vi "NanotecSMCPD.convert status.vi"(1 "status":T1 items=["motorEnabled"=1, "negativeLimitSwitchActive"=2, "positiveLimitSwitchActive"=4, "limitSwitchesEnabled"=8, "limitSwitchesAreNormallyClosed"=16, "moving"=32, "referenced"=64, "inPosition"=128, "reserved2"=256, "reserved3"=512, "reserved4"=1024, "reserved5"=2048, "error"=4096, "reserved6"=8192, "reserved7"=16384, "reserved8"=32768, "user defined1"=65536, "user defined2"=131072, "user defined3"=262144, "user defined4"=524288, "user defined5"=1048576, "user defined6"=2097152, "user defined7"=4194304, "user defined8"=8388608, "user defined9"=16777216, "user defined10"=33554432, "user defined11"=67108864, "user defined12"=134217728, "user defined13"=268435456, "user defined14"=536870912, "user defined15"=1073741824, "user defined16"=2147483648], 2 "actStatus type":T2) -> (15 "status out":T1 items=["motorEnabled"=1, "negativeLimitSwitchActive"=2, "positiveLimitSwitchActive"=4, "limitSwitchesEnabled"=8, "limitSwitchesAreNormallyClosed"=16, "moving"=32, "referenced"=64, "inPosition"=128, "reserved2"=256, "reserved3"=512, "reserved4"=1024, "reserved5"=2048, "error"=4096, "reserved6"=8192, "reserved7"=16384, "reserved8"=32768, "user defined1"=65536, "user defined2"=131072, "user defined3"=262144, "user defined4"=524288, "user defined5"=1048576, "user defined6"=2097152, "user defined7"=4194304, "user defined8"=8388608, "user defined9"=16777216, "user defined10"=33554432, "user defined11"=67108864, "user defined12"=134217728, "user defined13"=268435456, "user defined14"=536870912, "user defined15"=1073741824, "user defined16"=2147483648], 16 "motorOn":bool)   [LabVIEW 2014, in "NanotecSMCPD.lvlib"]
doc: "converts the status bytes received from the instrument driver to 32bit status word used by the MotorBase class."
uses:
  NanotecSMCPD.lvlib
  CSinstr.lib/NanotecSMCPD/Public/Action-Status/NanotecSMCPDDriver.status type.ctl
  CSCore/CSApplicationBaseClasses/MotorBase/MotorBase.statusType.ctl
  CSCore/CSApplicationBaseClasses/MotorBase/MotorBase.lvlib
  CSinstr.lib/NanotecSMCPD/NanotecSMCPDDriver.lvlib
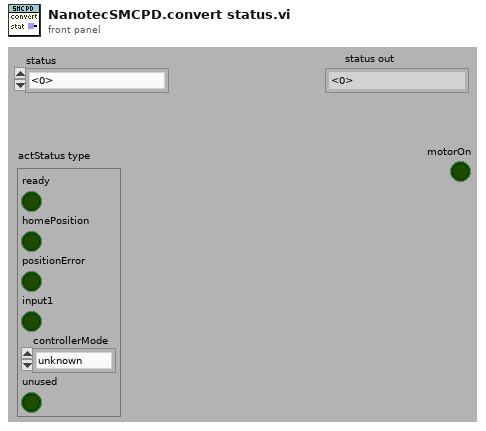
[diagram p1: front panel]
types:
  T1 = typedef "MotorBase.lvlib/MotorBase.statusType.ctl" = u32
  T2 = typedef "NanotecSMCPDDriver.lvlib/NanotecSMCPDDriver.status type.ctl" = cluster{"ready":bool, "homePosition":bool, "positionError":bool, "input1":bool, "controllerMode":enum16{"unknown", "position", "speed", "flagPosition", "clockDirection", "analog", "joystick", "unused"}, "unused":bool}
  T3 = enum16{"unknown", "position", "speed", "flagPosition", "clockDirection", "analog", "joystick", "unused"}
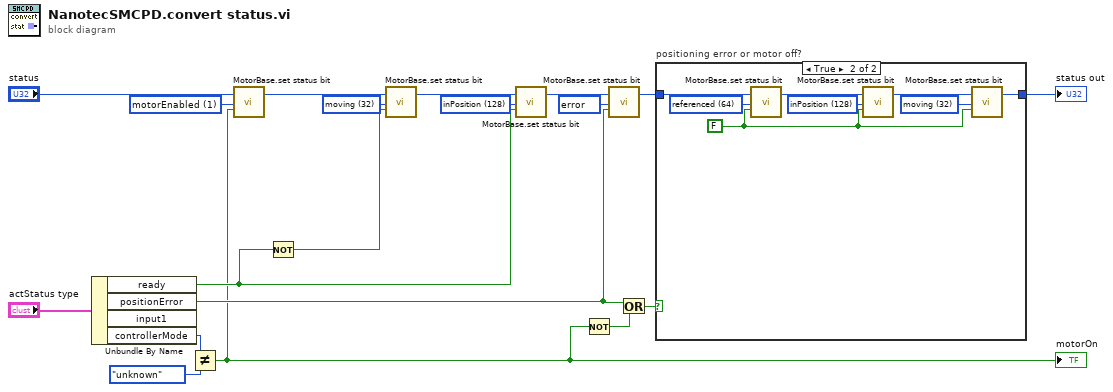
[diagram p0: block diagram]
diagram:
  w8 = T1 32 items=["motorEnabled"=1, "negativeLimitSwitchActive"=2, "positiveLimitSwitchActive"=4, "limitSwitchesEnabled"=8, "limitSwitchesAreNormallyClosed"=16, "moving"=32, "referenced"=64, "inPosition"=128, "reserved2"=256, "reserved3"=512, "reserved4"=1024, "reserved5"=2048, "error"=4096, "reserved6"=8192, "reserved7"=16384, "reserved8"=32768, "user defined1"=65536, "user defined2"=131072, "user defined3"=262144, "user defined4"=524288, "user defined5"=1048576, "user defined6"=2097152, "user defined7"=4194304, "user defined8"=8388608, "user defined9"=16777216, "user defined10"=33554432, "user defined11"=67108864, "user defined12"=134217728, "user defined13"=268435456, "user defined14"=536870912, "user defined15"=1073741824, "user defined16"=2147483648] ("statusBit")
  w15 = T1 4096 items=["motorEnabled"=1, "negativeLimitSwitchActive"=2, "positiveLimitSwitchActive"=4, "limitSwitchesEnabled"=8, "limitSwitchesAreNormallyClosed"=16, "reseved1"=32, "referenced"=64, "inPosition"=128, "reserved2"=256, "reserved3"=512, "reserved4"=1024, "reserved5"=2048, "error"=4096, "reserved6"=8192, "reserved7"=16384, "reserved8"=32768, "user defined1"=65536, "user defined2"=131072, "user defined3"=262144, "user defined4"=524288, "user defined5"=1048576, "user defined6"=2097152, "user defined7"=4194304, "user defined8"=8388608, "user defined9"=16777216, "user defined10"=33554432, "user defined11"=67108864, "user defined12"=134217728, "user defined13"=268435456, "user defined14"=536870912, "user defined15"=1073741824, "user defined16"=2147483648] ("statusBit")
  w16 = T1 128 items=["motorEnabled"=1, "negativeLimitSwitchActive"=2, "positiveLimitSwitchActive"=4, "limitSwitchesEnabled"=8, "limitSwitchesAreNormallyClosed"=16, "reseved1"=32, "referenced"=64, "inPosition"=128, "reserved2"=256, "reserved3"=512, "reserved4"=1024, "reserved5"=2048, "error"=4096, "reserved6"=8192, "reserved7"=16384, "reserved8"=32768, "user defined1"=65536, "user defined2"=131072, "user defined3"=262144, "user defined4"=524288, "user defined5"=1048576, "user defined6"=2097152, "user defined7"=4194304, "user defined8"=8388608, "user defined9"=16777216, "user defined10"=33554432, "user defined11"=67108864, "user defined12"=134217728, "user defined13"=268435456, "user defined14"=536870912, "user defined15"=1073741824, "user defined16"=2147483648] ("statusBit")
  w17 = T1 1 items=["motorEnabled"=1, "negativeLimitSwitchActive"=2, "positiveLimitSwitchActive"=4, "limitSwitchesEnabled"=8, "limitSwitchesAreNormallyClosed"=16, "reseved1"=32, "referenced"=64, "inPosition"=128, "reserved2"=256, "reserved3"=512, "reserved4"=1024, "reserved5"=2048, "error"=4096, "reserved6"=8192, "reserved7"=16384, "reserved8"=32768, "user defined1"=65536, "user defined2"=131072, "user defined3"=262144, "user defined4"=524288, "user defined5"=1048576, "user defined6"=2097152, "user defined7"=4194304, "user defined8"=8388608, "user defined9"=16777216, "user defined10"=33554432, "user defined11"=67108864, "user defined12"=134217728, "user defined13"=268435456, "user defined14"=536870912, "user defined15"=1073741824, "user defined16"=2147483648] ("statusBit")
  n1 = Unbundle By Name("actStatus type") -> ("ready"=w5:bool, "positionError"=w4:bool, "controllerMode"=w13:T3)  [unwired: 1 out]
  n2 = Not Equal?(x=w13, y=T3."unknown" ("controllerMode")) -> (x != y?=w2:bool)
  "motorOn" <- w2
  n3 = call "MotorBase.set status bit.vi"("status"="status", "statusBit"=w17, "setBit"=w2) -> ("status out"=w11:T1)  [unwired: 16 in]
  n4 = Not(x=w5) -> (.not. x?=w9:bool)
  n5 = call "MotorBase.set status bit.vi"("status"=w11, "statusBit"=w8, "setBit"=w9) -> ("status out"=w10:T1)  [unwired: 16 in]
  n6 = call "MotorBase.set status bit.vi"("status"=w10, "statusBit"=w16, "setBit"=w5) -> ("status out"=w12:T1)  [unwired: 16 in]
  n7 = Not(x=w2) -> (.not. x?=w1:bool)
  n8 = call "MotorBase.set status bit.vi"("status"=w12, "statusBit"=w15, "setBit"=w4) -> ("status out"=w7:T1)  [unwired: 16 in]
  n9 = Or(x=w4, y=w1) -> (x .or. y?=w3:bool)
  n10 = case "positioning error or motor off?" shown="True" w3 {
    tunnel: w7 -> [w20 w28]
    tunnel: [w20 w23] -> w6
    frame False {
    }
    frame True {
      w22 = T1 32 items=["motorEnabled"=1, "negativeLimitSwitchActive"=2, "positiveLimitSwitchActive"=4, "limitSwitchesEnabled"=8, "limitSwitchesAreNormallyClosed"=16, "moving"=32, "referenced"=64, "inPosition"=128, "reserved2"=256, "reserved3"=512, "reserved4"=1024, "reserved5"=2048, "error"=4096, "reserved6"=8192, "reserved7"=16384, "reserved8"=32768, "user defined1"=65536, "user defined2"=131072, "user defined3"=262144, "user defined4"=524288, "user defined5"=1048576, "user defined6"=2097152, "user defined7"=4194304, "user defined8"=8388608, "user defined9"=16777216, "user defined10"=33554432, "user defined11"=67108864, "user defined12"=134217728, "user defined13"=268435456, "user defined14"=536870912, "user defined15"=1073741824, "user defined16"=2147483648] ("statusBit")
      w25 = T1 128 items=["motorEnabled"=1, "negativeLimitSwitchActive"=2, "positiveLimitSwitchActive"=4, "limitSwitchesEnabled"=8, "limitSwitchesAreNormallyClosed"=16, "moving"=32, "referenced"=64, "inPosition"=128, "reserved2"=256, "reserved3"=512, "reserved4"=1024, "reserved5"=2048, "error"=4096, "reserved6"=8192, "reserved7"=16384, "reserved8"=32768, "user defined1"=65536, "user defined2"=131072, "user defined3"=262144, "user defined4"=524288, "user defined5"=1048576, "user defined6"=2097152, "user defined7"=4194304, "user defined8"=8388608, "user defined9"=16777216, "user defined10"=33554432, "user defined11"=67108864, "user defined12"=134217728, "user defined13"=268435456, "user defined14"=536870912, "user defined15"=1073741824, "user defined16"=2147483648] ("statusBit")
      w21 = FALSE ("setBit")
      w27 = T1 64 items=["motorEnabled"=1, "negativeLimitSwitchActive"=2, "positiveLimitSwitchActive"=4, "limitSwitchesEnabled"=8, "limitSwitchesAreNormallyClosed"=16, "moving"=32, "referenced"=64, "inPosition"=128, "reserved2"=256, "reserved3"=512, "reserved4"=1024, "reserved5"=2048, "error"=4096, "reserved6"=8192, "reserved7"=16384, "reserved8"=32768, "user defined1"=65536, "user defined2"=131072, "user defined3"=262144, "user defined4"=524288, "user defined5"=1048576, "user defined6"=2097152, "user defined7"=4194304, "user defined8"=8388608, "user defined9"=16777216, "user defined10"=33554432, "user defined11"=67108864, "user defined12"=134217728, "user defined13"=268435456, "user defined14"=536870912, "user defined15"=1073741824, "user defined16"=2147483648] ("statusBit")
      n11 = call "MotorBase.set status bit.vi"("status"=w28, "statusBit"=w27, "setBit"=w21) -> ("status out"=w26:T1)  [unwired: 16 in]
      n12 = call "MotorBase.set status bit.vi"("status"=w26, "statusBit"=w25, "setBit"=w21) -> ("status out"=w24:T1)  [unwired: 16 in]
      n13 = call "MotorBase.set status bit.vi"("status"=w24, "statusBit"=w22, "setBit"=w21) -> ("status out"=w23:T1)  [unwired: 16 in]
    }
  }
  "status out" <- w6
